vi "AddCondiments.vi"(8 "error in (no error)":errorcluster, 11 "Coffee in":refnum<class "Coffee.lvclass">) -> (0 "error out":errorcluster, 2 "ProcessMessage":string, 3 "Coffee out":refnum<class "Coffee.lvclass">)   [LabVIEW 2013, in "Coffee.lvclass"]
uses:
  Coffee.lvclass
  CaffeineBeverage.lvclass/CaffeineBeverage.lvclass
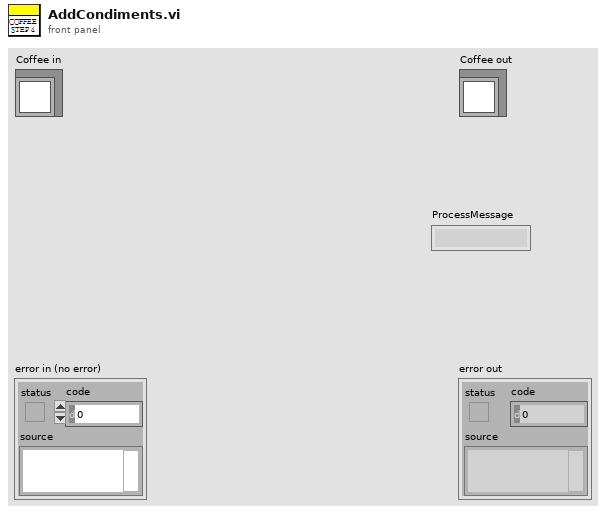
[diagram p1: front panel]
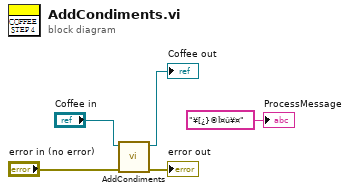
[diagram p0: block diagram]
diagram:
  n1 = call-parent "AddCondiments.vi"("error in (no error)"="error in (no error)", "CaffeineBeverage in"="Coffee in") -> ("error out"=→"error out":errorcluster, "CaffeineBeverage out"=→"Coffee out":refnum<class "Coffee.lvclass">)  [unwired: 7 in, 1 out]
  "ProcessMessage" <- "¥[¿}©Î¤û¥¤" ("ProcessMessage")
